vi "Calculation Distance.vi"(8 "error in":errorcluster caption="error out") -> (0 "error out":errorcluster caption="error in")   [LabVIEW 2015, in "Debug.lvlib"]
uses:
  Debug.lvlib
  Support/Calculation Distance State.ctl
  <vilib>/vision/Image Controls.llb/IMAQ Image.ctl
  Sub VIs/Digital Image Processing/Support/Ellipse.ctl
  Sub VIs/Utility VIs/Utility VIs.lvlib
  Sub VIs/Digital Image Processing/Digital Image Processing.lvlib
panel:
  in  "停止按钮":bool
  out "平均距离":dbl
  out "外圆距离":dbl
  out "内圆距离":dbl
  out "Image":T1(plugin-control)
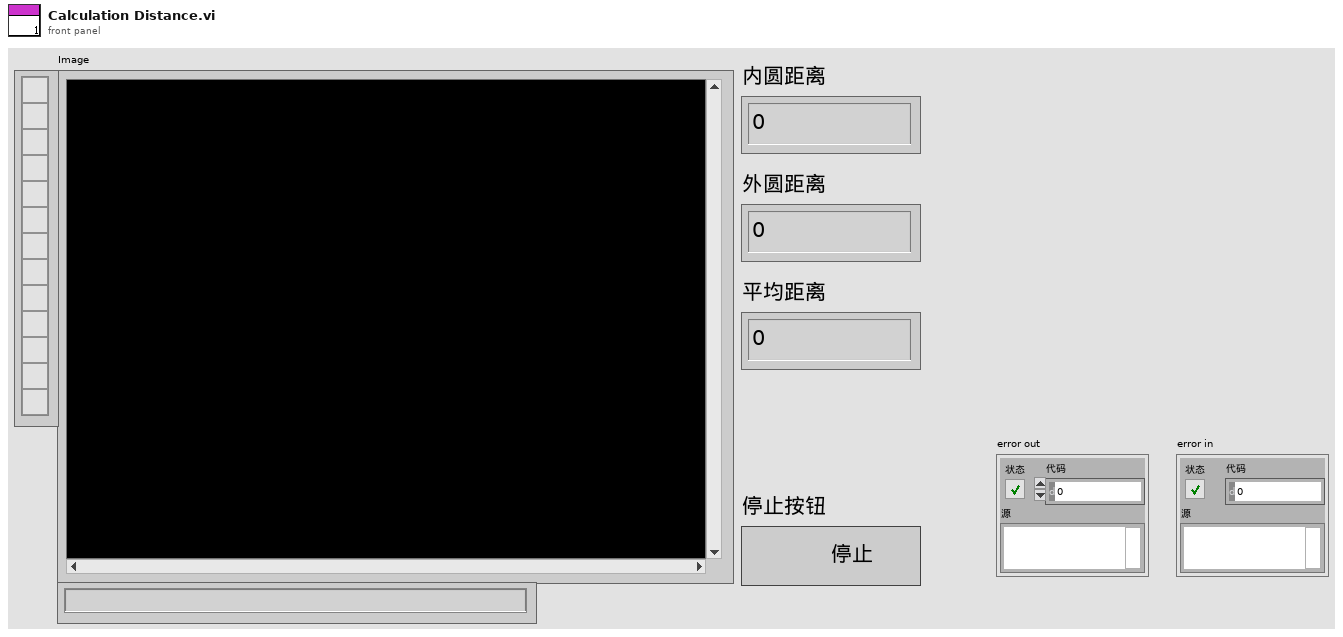
[diagram p1: front panel]
types:
  T1 = typedef "IMAQ Image.ctl" = refnum<image>
  T2 = typedef "Debug.lvlib/Calculation Distance State.ctl" = enum16{"Initialize", "Load Image", "Calculation", "Save", "Wait For Event", "Exit"}
  T3 = typedef "Digital Image Processing.lvlib/Ellipse.ctl" = cluster{"A":dbl, "B":dbl, "x0":dbl, "y0":dbl, "phi":dbl}
  T4 = cluster{"A":dbl, "B":dbl, "x0":dbl, "y0":dbl, "phi":dbl}
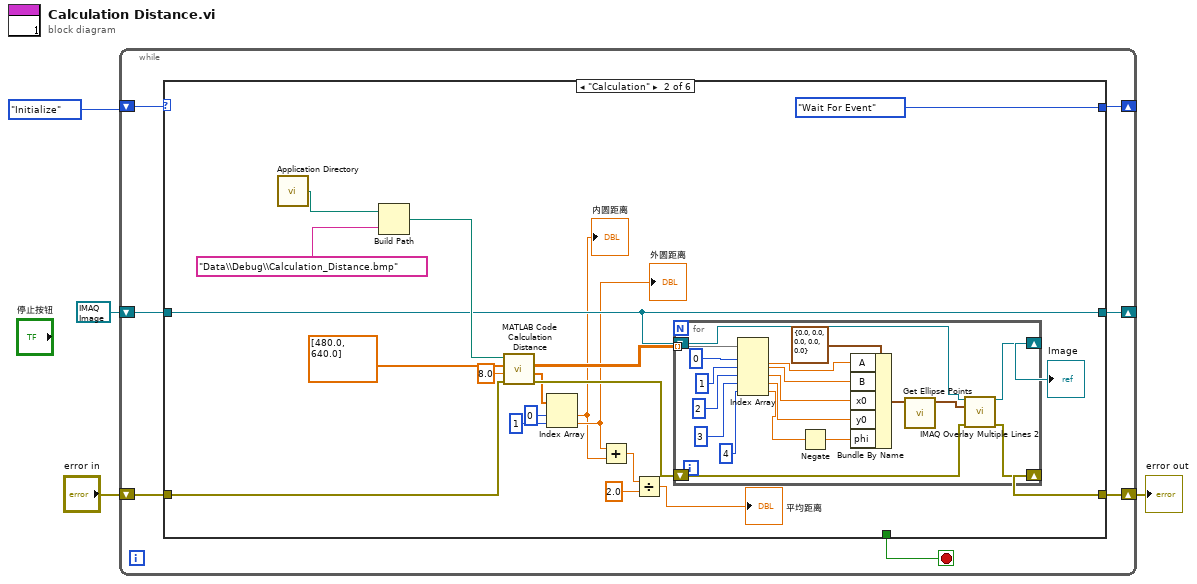
[diagram p0: block diagram]
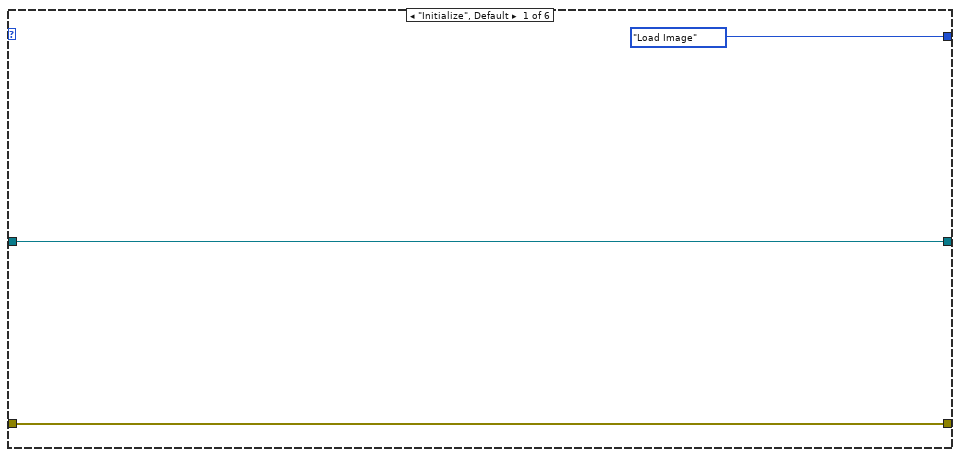
[diagram p2: hidden frame]
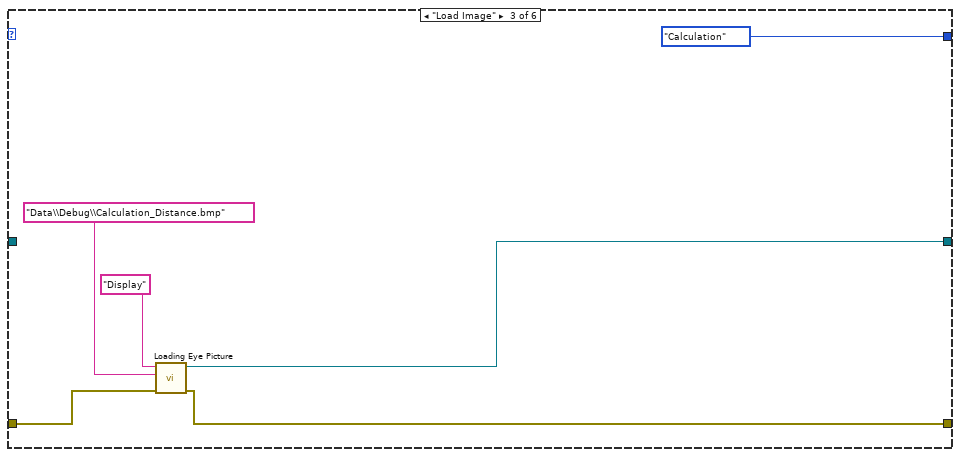
[diagram p3: hidden frame]
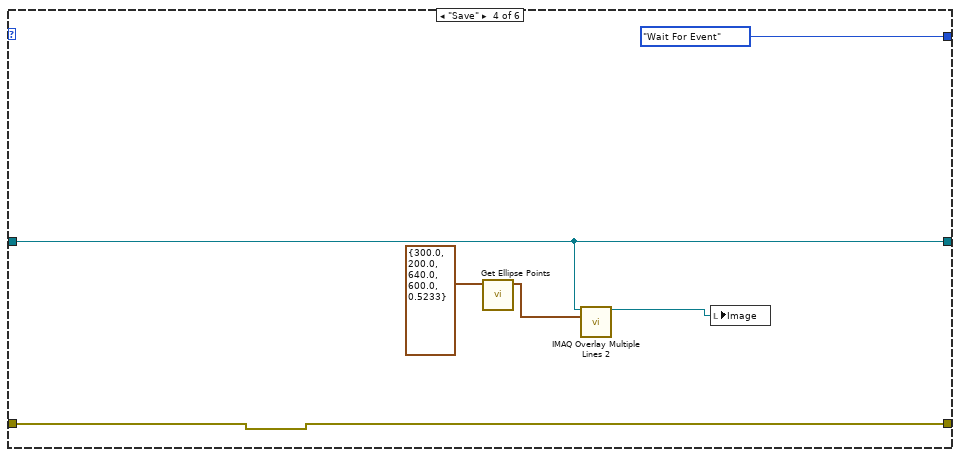
[diagram p4: hidden frame]
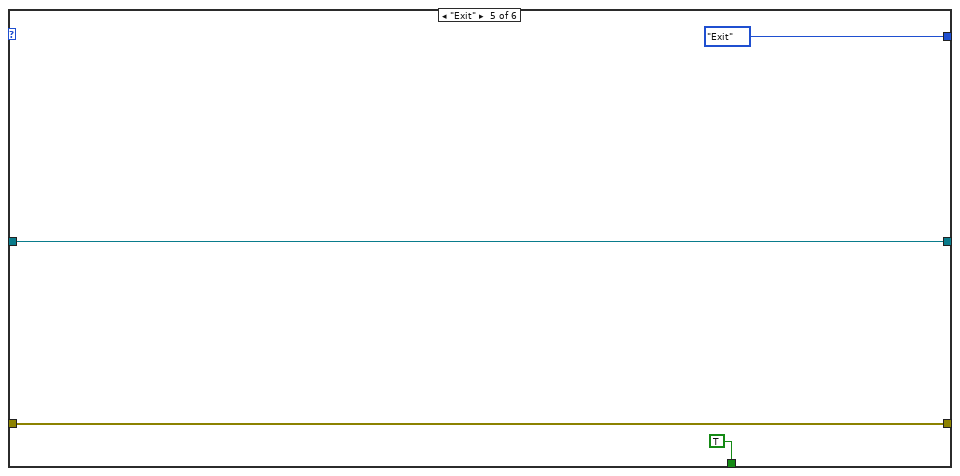
[diagram p5: hidden frame]
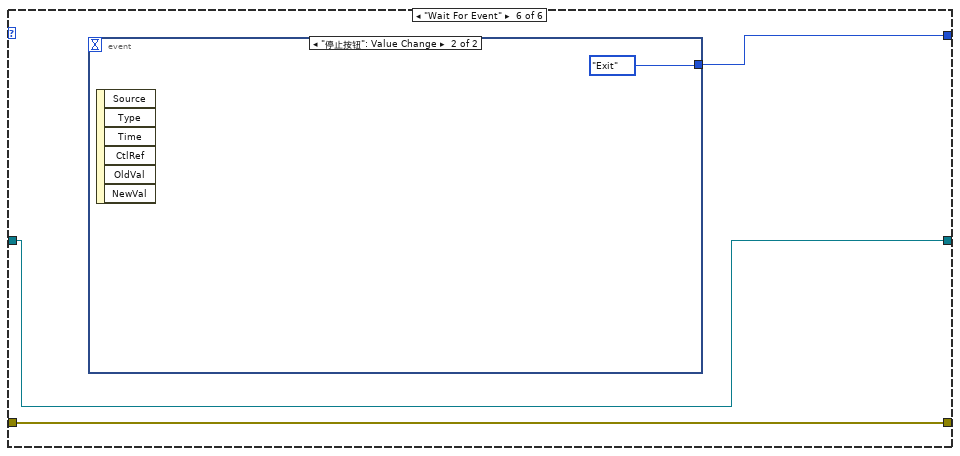
[diagram p6: hidden frame]
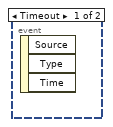
[diagram p7: hidden frame]
diagram:
  n1 = while {
    shift-right: [w10] -> _
    shift-left: Calculation_Distance_State."Initialize" ("Calculation Distance State") -> [w11]
    shift-right: [w8] -> w1
    shift-left: "error in" -> [w7]
    shift-right: [w6] -> _
    shift-left: T1 refnum ("Image Out") -> [w5]
    stop <- w9 stop-if-true
    n2 = case shown="\"Calculation\"" w11 {
      tunnel: [Calculation_Distance_State."Load Image" ("Calculation Distance State") Calculation_Distance_State."Wait For Event" ("Calculation Distance State") Calculation_Distance_State."Calculation" ("Calculation Distance State") Calculation_Distance_State."Wait For Event" ("Calculation Distance State") Calculation_Distance_State."Exit" ("Calculation Distance State") w72] -> w10
      tunnel: [_ _ _ _ TRUE _] -> w9
      tunnel: w7 -> [w12 w28 w58 w64 w66 w70]
      tunnel: [w12 w23 w57 w64 w66 w70] -> w8
      tunnel: [w13 w25 w54 w61 w67 w71] -> w6
      tunnel: w5 -> [w13 w25 _ w61 w67 w71]
      frame "Initialize", Default {
      }
      frame "Calculation" {
        n3 = call <vilib>:"Application Directory.vi"() -> ("Application Directory"=w33:path)
        n4 = Build Path(base path=w33, name or relative path="Data\\Debug\\Calculation_Distance.bmp" ("名称或相对路径")) -> (appended path=w31:path)
        n5 = call "MATLAB Code Calculation Distance.vi"("error in (no error)"=w28, "R"=8.0, "centre"=dbl[] [480.0, 640.0], "Path"=w31) -> ("error out"=w26:errorcluster, "Distance"=w22:dbl[], "Ellipse"=w27:dbl[][])  [unwired: 4 in, 1 out]
        n6 = Index Array(array=w22, index #1=0 ("索引"), index #2=1 ("索引")) -> (element #1=w18:dbl, element #2=w19:dbl)
        "内圆距离" <- w18
        "外圆距离" <- w19
        n7 = Add(x=w19, y=w18) -> (x+y=w17:dbl)
        n8 = Divide(x=w17, y=2.0) -> (x/y=→"平均距离":dbl)
        n9 = for {
          tunnel: w27 -> [w53] mode=indexing
          shift-right: [w39] -> w23
          shift-left: w26 -> [w40]
          shift-right: [w37] -> w24
          shift-left: w25 -> [w38]
          n10 = Index Array(array=w53, index #1=0 ("索引"), index #2=1 ("索引"), index #3=2 ("索引"), index #4=3 ("索引"), index #5=4 ("索引")) -> (element #1=w46:dbl, element #2=w45:dbl, element #3=w44:dbl, element #4=w43:dbl, element #5=w35:dbl)
          n11 = Negate(x=w35) -> (-x=w36:dbl)
          n12 = Bundle By Name(cluster=T3 {"A"=0.0, "B"=0.0, "x0"=0.0, "y0"=0.0, "phi"=0.0} ("Ellipse"), "A"=w46, "B"=w45, "x0"=w44, "y0"=w43, "phi"=w36) -> (w42:T3)
          n13 = call "Get Ellipse Points.vi"("Ellipse"=w42) -> ("Points"=w41:cluster{dbl, dbl}[])  [unwired: 10 in]
          n14 = call "IMAQ Overlay Multiple Lines 2"("Image"=w38, "Line End Points"=w41, "error in (no error)"=w40) -> ("Image Out"=w37:T1, "error out"=w39:errorcluster)  [unwired: 11 in]
        }
        "Image" <- w24
      }
      frame "Load Image" {
        n15 = call "Loading Eye Picture.vi"("error in (no error)"=w58, "名称或相对路径"="Data\\Debug\\Calculation_Distance.bmp", "Image Name"="Display") -> ("error out"=w57:errorcluster, "Image Out"=w54:T1)  [unwired: 7 in]
      }
      frame "Save" {
        n16 = call "Get Ellipse Points.vi"("Ellipse"=T4 {"A"=300.0, "B"=200.0, "x0"=640.0, "y0"=600.0, "phi"=0.5233}) -> ("Points"=w62:cluster{dbl, dbl}[])  [unwired: 10 in]
        n17 = call "IMAQ Overlay Multiple Lines 2"("Image"=w61, "Line End Points"=w62) -> ("Image Out"=w60:T1)  [unwired: 12 in, 1 out]
        n18 = local write "Image"(w60) -> ()
      }
      frame "Exit" {
      }
      frame "Wait For Event" {
        n19 = event shown="[1] \"停止按钮\": Value Change" {
          selector: _ -> [_ _]
          dyn-events: _ -> [_ _]
          timeout: _ -> [_ _]
          tunnel: [_ Calculation_Distance_State."Exit" ("Calculation Distance State")] -> w72
          event Timeout {
            n20 = event-data() -> ()  [unwired: 1 in, 3 out]
          }
          event "停止按钮": Value Change {
            n21 = event-data() -> ()  [unwired: 1 in, 6 out]
          }
        }
      }
    }
  }
  "error out" <- w1
